vi "Set_DIO_Config.vi"(4 "#DescreteOutputs":u16, 6 "#DescreteInputs":u16, 8 "error in (no error)":errorcluster, 9 "StartAddress_DO":u16, 10 "StartAddress_DI":u16, 11 "Device in":refnum<class "DAQ_Device.lvclass">) -> (0 "error out":errorcluster, 3 "Device out":refnum<class "DAQ_Device.lvclass">)   [LabVIEW 2023, in "DAQ_Device.lvclass"]
uses:
  DAQ_Device.lvclass
  DAQ_Device.lvclass/DAQ_Device.ctl
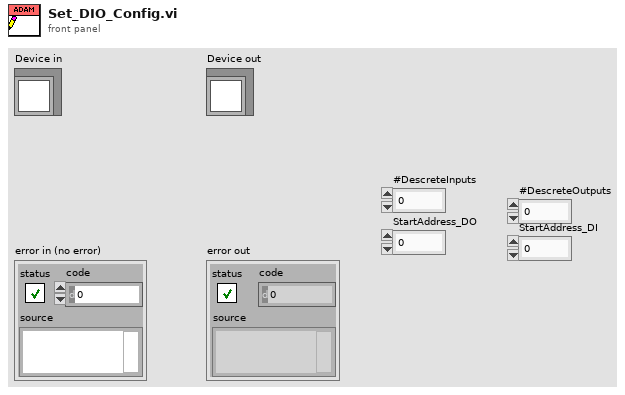
[diagram p1: front panel]
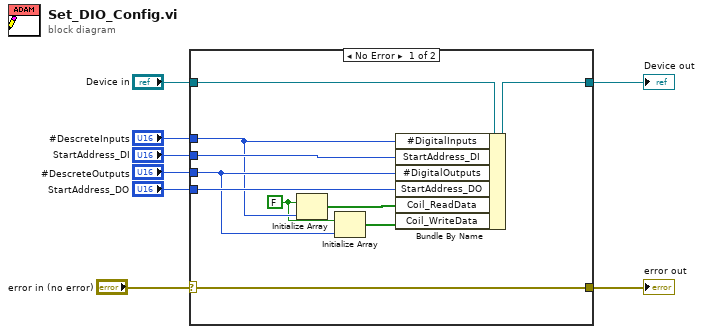
[diagram p0: block diagram]
diagram:
  n1 = case shown="No Error" "error in (no error)" {
    selector: "error in (no error)" -> [w12 w19]
    tunnel: [w12 w19] -> w7
    tunnel: [w17 w20] -> w5
    tunnel: "Device in" -> [w18 w20]
    tunnel: "StartAddress_DO" -> [w16 _]
    tunnel: "StartAddress_DI" -> [w15 _]
    tunnel: "#DescreteOutputs" -> [w14 _]
    tunnel: "#DescreteInputs" -> [w13 _]
    frame No Error {
      w9 = FALSE
      n2 = Initialize Array(w9, w13) -> (w11:bool[])
      n3 = Initialize Array(w9, w14) -> (w10:bool[])
      n4 = Bundle By Name(cluster=w18, "#DigitalInputs"=w13, "StartAddress_DI"=w15, "#DigitalOutputs"=w14, "StartAddress_DO"=w16, "Coil_ReadData"=w11, "Coil_WriteData"=w10) -> (w17:refnum<class "DAQ_Device.lvclass">)
    }
    frame Error {
    }
  }
  "error out" <- w7
  "Device out" <- w5
